vi "SubVI2.vi"(10 "B":dbl[](array[numeric]), 11 "A":dbl[](array[numeric])) -> (2 "B 2":dbl[](array[numeric]), 3 "A 2":dbl[](array[numeric]))   [LabVIEW 2011]
doc: "This VI adds and subtracts two arrays"
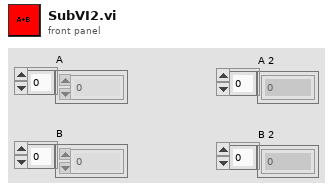
[diagram p1: front panel]
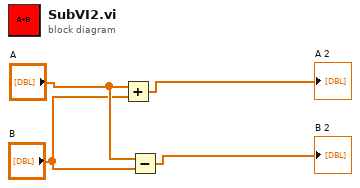
[diagram p0: block diagram]
diagram:
  n1 = Add(x="A", y="B") -> (x+y=→"A 2":dbl[])
  n2 = Subtract(x="A", y="B") -> (x-y=→"B 2":dbl[])
